vi "ITR HP order 3.vi"(7 "input":dbl format="%.2f", 13 "corner period (steps)":dbl(slide)=10.237739663395852 scale=1.0..1000.0) -> (8 "output":dbl format="%.2f")   [LabVIEW 2016]
doc: "Modular ITR third order high pass filter with internal shift registers.\n\nAlexis Lopez\nP350\nCSUSB Physics"
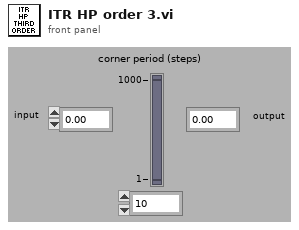
[diagram p1: front panel]
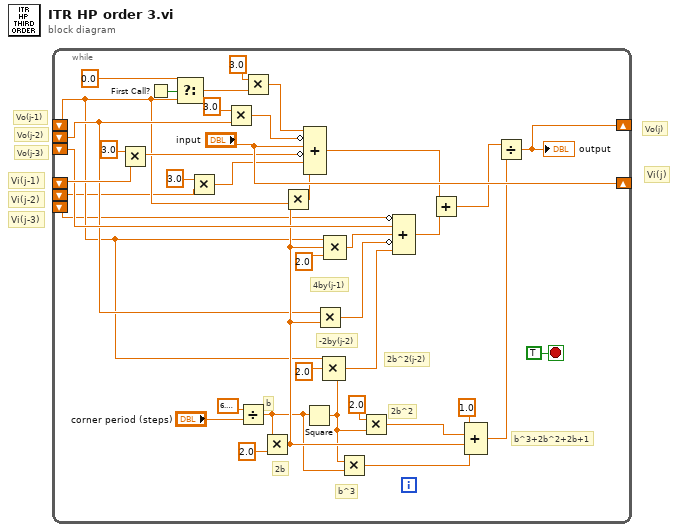
[diagram p0: block diagram]
diagram:
  # "Vi(j-3)"
  # "Vo(j-3)"
  # "Vo(j-2)"
  # "Vi(j-2)"
  # "Vi(j-1)"
  # "Vi(j)"
  # "Vo(j-1)"
  # "Vo(j)"
  n1 = while {
    shift-left: _ -> [w14]
    shift-right: [w37] -> _
    shift-right: ["input"] -> _
    shift-left: _ -> [w33]
    shift-left: _ -> [w17]
    shift-left: _ -> [w11]
    shift-left: _ -> [w22]
    shift-left: _ -> [w9]
    stop <- TRUE stop-if-true
    # "b^3"
    # "2b^2(j-2)"
    # "-2by(j-2)"
    # "4by(j-1)"
    # "2b^2"
    # "2b"
    # "b^3+2b^2+2b+1"
    # "b"
    n2 = Multiply(x=3.0, y=w33) -> (x*y=w31:dbl)
    n3 = First Call?() -> (First Call?: T/F=w36:bool)
    n4 = Select(t=0.0, s=w36, f=w14) -> (s? t:f=w30:dbl)
    n5 = Multiply(x=3.0, y=w11) -> (x*y=w10:dbl)
    n6 = Multiply(x=3.0, y=w17) -> (x*y=w23:dbl)
    n7 = Divide(x=6.283185307179586, y="corner period (steps)") -> (x/y=w3:dbl)
    n8 = Multiply(x=3.0, y=w30) -> (x*y=w28:dbl)
    n9 = Multiply(x=w3, y=2.0) -> (x*y=w18:dbl)
    n10 = Multiply(x=w14, y=w18) -> (x*y=w25:dbl)
    n11 = Compound Arithmetic op=ADD(w28, invert w23, "input", invert w31, w10, w25) -> (w7:dbl)
    n12 = Square(x=w3) -> (x^2=w2:dbl)
    n13 = Multiply(x=w17, y=w18) -> (x*y=w16:dbl)
    n14 = Compound Arithmetic op=MULTIPLY(w14, 2.0, w2) -> (w13:dbl)
    n15 = Compound Arithmetic op=MULTIPLY(w14, w18, 2.0) -> (w19:dbl)
    n16 = Multiply(x=w2, y=w3) -> (x*y=w1:dbl)
    n17 = Multiply(x=2.0, y=w2) -> (x*y=w4:dbl)
    n18 = Compound Arithmetic op=ADD(invert w9, w22, w19, invert w16, w13) -> (w8:dbl)
    n19 = Add(x=w7, y=w8) -> (x+y=w6:dbl)
    n20 = Compound Arithmetic op=ADD(1.0 ("t"), w4, w18, w1) -> (w26:dbl)
    n21 = Divide(x=w6, y=w26) -> (x/y=w37:dbl)
    "output" <- w37
  }
